vi "mask lineout.vi"(9 "X Axis Averages":dbl[](graph), 10 "half width for 2nd mom cut":sgl, 11 "X Centroid":sgl) -> (2 "updated centroid":dbl, 3 "Waveform Graph":dbl[](graph))   [LabVIEW 2020]
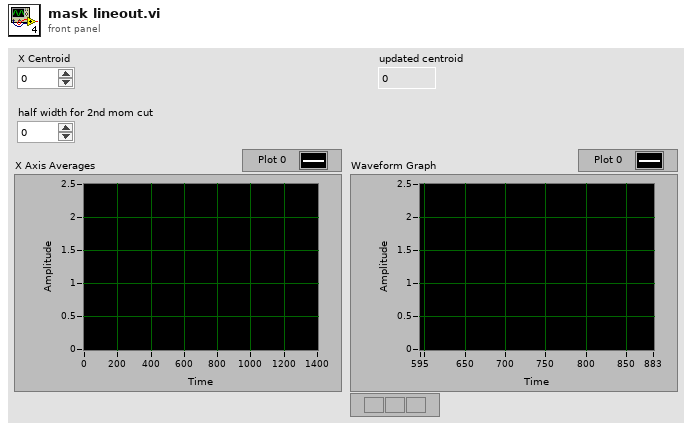
[diagram p1: front panel]
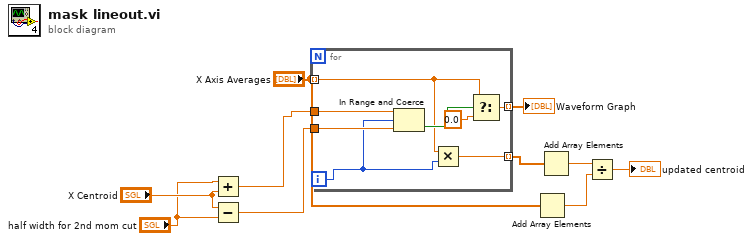
[diagram p0: block diagram]
diagram:
  n1 = Add(x="half width for 2nd mom cut", y="X Centroid") -> (x+y=w7:sgl)
  n2 = Subtract(x="X Centroid", y="half width for 2nd mom cut") -> (x-y=w6:sgl)
  n3 = for {
    tunnel: "X Axis Averages" -> [w13] mode=indexing
    tunnel: [w16] -> w10 mode=indexing
    tunnel: w7 -> [w15]
    tunnel: w6 -> [w14]
    tunnel: [w11] -> w5 mode=indexing
    i -> [w12]
    n4 = In Range and Coerce(upper limit=w15, x=w12, lower limit=w14) -> (In Range?=w18:bool)  [unwired: 1 out]
    n5 = Multiply(x=w13, y=w12) -> (x*y=w11:dbl)
    n6 = Select(t=w13, s=w18, f=sgl 0.0) -> (s? t:f=w16:dbl)
  }
  "Waveform Graph" <- w10
  n7 = Add Array Elements(numeric array="X Axis Averages") -> (sum=w2:dbl)
  n8 = Add Array Elements(numeric array=w5) -> (sum=w4:dbl)
  n9 = Divide(x=w4, y=w2) -> (x/y=→"updated centroid":dbl)
